vi "SensorTester.vi"() -> ()   [LabVIEW 2019]
uses:
  <vilib>/myRIO/Instrument Drivers/Onboard IO/AI/typedefs/AI Reference.ctl
  <vilib>/myRIO/Common/Instrument Driver Framework/Utilities/typedefs/myRIO Generic Hardware Reference.ctl
  <vilib>/myRIO/Common/Instrument Driver Framework/Utilities/typedefs/Hardware Version Enum.ctl
  <vilib>/myRIO/Common/Instrument Driver Framework/Utilities/typedefs/myRIO v1.0 Reference.ctl
  <vilib>/myRIO/Common/Instrument Driver Framework/Utilities/typedefs/Generic FPGA Reference.ctl
  <vilib>/myRIO/Common/Instrument Driver Framework/myRIO v1.0/AI/typedefs/AI Channels List.ctl
  <vilib>/myRIO/Common/Instrument Driver Framework/myRIO v1.0/AI/typedefs/AI Channels Enum.ctl
  <vilib>/myRIO/Common/Instrument Driver Framework/Utilities/typedefs/Analog Scaling Constants List.ctl
  <vilib>/myRIO/Common/Instrument Driver Framework/Utilities/typedefs/Analog Scaling Constants.ctl
  <vilib>/userDefined/High Color/nirio_resource_hc.ctl
  <vilib>/myRIO/Instrument Drivers/Onboard IO/PWM/typedefs/PWM Reference.ctl
  <vilib>/myRIO/Common/Instrument Driver Framework/myRIO v1.0/PWM/typedefs/PWM Channels Enum.ctl
  <vilib>/myRIO/Instrument Drivers/Onboard IO/PWM/typedefs/PWM Configuration.ctl
  <vilib>/myRIO/Common/Instrument Driver Framework/Utilities/vis/Is FPGA Ref Available.vi
  <vilib>/myRIO/Common/Instrument Driver Framework/myRIO v1.0/AI/vis/myRIO v1.1 Open AI.vi
  <vilib>/myRIO/Instrument Drivers/Onboard IO/AI/vis/Read.vi
  <vilib>/myRIO/Common/Instrument Driver Framework/myRIO v1.0/PWM/vis/myRIO v1.1 Open PWM.vi
  <vilib>/myRIO/Instrument Drivers/Onboard IO/PWM/vis/Set Duty Cycle and Frequency.vi
  <vilib>/myRIO/Common/Instrument Driver Framework/Utilities/vis/Validate Channels.vi
  <vilib>/myRIO/Common/Instrument Driver Framework/myRIO v1.0/AI/vis/myRIO v1.0 Reserve AI.vi
  <vilib>/myRIO/Common/Instrument Driver Framework/myRIO v1.0/PWM/vis/myRIO v1.0 Reserve PWM.vi
  <vilib>/myRIO/Common/Instrument Driver Framework/myRIO v1.0/UART/vis/myRIO v1.0 Close UART.vi
  <vilib>/myRIO/Common/Instrument Driver Framework/myRIO v1.0/AI/vis/myRIO v1.0 Build MUX Configuration AI.vi
  <vilib>/myRIO/Common/Instrument Driver Framework/myRIO v1.0/Resource Manager/vis/myRIO v1.0 Reserve Channel List.vi
  <vilib>/myRIO/Common/Instrument Driver Framework/myRIO v1.0/PWM/vis/myRIO v1.0 Build MUX Configuration PWM.vi
  <vilib>/myRIO/Common/Instrument Driver Framework/myRIO v1.0/Resource Manager/vis/myRIO v1.0 Reserve Channel.vi
  <vilib>/myRIO/Common/Instrument Driver Framework/myRIO v1.0/Resource Manager/vis/myRIO v1.0 Unreserve Channel.vi
  <vilib>/myRIO/Common/Instrument Driver Framework/myRIO v1.0/Resource Manager/vis/myRIO v1.0 Create Configuration List.vi
  <vilib>/myRIO/Common/Instrument Driver Framework/myRIO v1.0/Resource Manager/vis/myRIO v1.0 Build Mutex Name.vi
  <vilib>/Utility/VariantDataType/GetNumericInfo.vi
  <vilib>/Utility/error.llb/Error Cluster From Error Code.vi
  <vilib>/myRIO/Common/Instrument Driver Framework/myRIO v1.0/myRIO v1.1 Open.vi
  <vilib>/myRIO/Common/Instrument Driver Framework/myRIO v1.0/AI/vis/myRIO v1.0 Get Scaling Constants AI.vi
  <vilib>/myRIO/Common/Instrument Driver Framework/Utilities/vis/IO Manager.vi
  <vilib>/myRIO/Common/Instrument Driver Framework/Utilities/vis/Configuration Manager.vi
  <vilib>/myRIO/Common/Instrument Driver Framework/myRIO v1.0/myRIO v1.0 Close.vi
  <vilib>/myRIO/Common/Instrument Driver Framework/myRIO v1.0/AI/vis/myRIO v1.0 Read AI.vi
  <vilib>/imath/engines/lvmath2/RunTimeEngine/Managers/WorkSpace/UID Generator.vi
  <vilib>/imath/engines/lvmath2/RunTimeEngine/RunTimeType/NIMS_RunTimeType_From StrictType (excl LVString).vi
  <instcachedir>/0/NIMS_RunTimeType_From StrictType (excl LVString)_D8AFBA86A94845AAA577C895450664BD.lvgen/NIMS_RunTimeType_From StrictType (excl LVString)_D8AFBA86A94845AAA577C895450664BD_000.vi
  <vilib>/imath/engines/lvmath2/RunTimeEngine/LocalVariableDefStatement/MC_LocalVariableDefStatement_Display.vi
  <vilib>/imath/engines/lvmath2/RunTimeEngine/Managers/SymbolTable/Clear UID.vi
  <vilib>/imath/engines/lvmath2/RunTimeEngine/NodeEndStatement/NIMS_NodeEndStatement_Output.vi
  <instcachedir>/0/NIMS_NodeEndStatement_Output_53EC0D466D134D7ABD903AC30B43404B.lvgen/NIMS_NodeEndStatement_Output_53EC0D466D134D7ABD903AC30B43404B_001.vi
  <vilib>/imath/engines/lvmath2/RunTimeEngine/ErrorHandling/NIMS_Finalize Error.vi
  <vilib>/addons/control/pid/pid.llb/PID (DBL).vi
  <vilib>/myRIO/Common/Instrument Driver Framework/myRIO v1.0/Resource Manager/vis/myRIO v1.0 Configure IO.vi
  <vilib>/myRIO/Common/Instrument Driver Framework/myRIO v1.0/PWM/vis/myRIO v1.0 Write PWM.vi
  <vilib>/myRIO/Common/Instrument Driver Framework/Utilities/vis/FPGA Ref Manager.vi
  <vilib>/myRIO/Common/Instrument Driver Framework/myRIO v1.0/myRIO v1.0 Reset FPGA.vi
  <vilib>/myRIO/Common/Instrument Driver Framework/myRIO v1.0/IRQ/vis/myRIO v1.0 IRQ Info FGV.vi
  <vilib>/myRIO/Common/Instrument Driver Framework/myRIO v1.0/IRQ/vis/myRIO v1.0 Timer IRQ Info FGV.vi
  <vilib>/myRIO/Common/Instrument Driver Framework/myRIO v1.0/IRQ/vis/myRIO v1.0 ISR Agent.vi
  <vilib>/myRIO/Instrument Drivers/Utilities/vis/Reset Index.vi
  <vilib>/myRIO/Common/Instrument Driver Framework/myRIO v1.0/Resource Manager/vis/myRIO v1.0 Block Write Resource Manager.vi
  <vilib>/myRIO/Express VI/Onboard IO/AI/AI Express VI.xnode
  <vilib>/myRIO/Instrument Drivers/Onboard IO/AI/vis/myRIO AI Open.xnode
  <vilib>/myRIO/Express VI/Onboard IO/PWM/PWM Express VI.xnode
  <vilib>/myRIO/Instrument Drivers/Onboard IO/PWM/vis/myRIO PWM Open.xnode
  <vilib>/myRIO/Instrument Drivers/Onboard IO/PWM/PWM.lvlib
  <vilib>/myRIO/Instrument Drivers/Onboard IO/AI/AI.lvlib
  <vilib>/imath/engines/lvmath2/RunTimeEngine/Managers/SymbolTable/NIMS_WorkSpace.lvlib
  <vilib>/addons/control/pid/NI_PID_pid.lvlib
  <vilib>/ptbypt/NI_PtbyPt.lvlib
  <vilib>/myRIO/Instrument Drivers/Utilities/Utilities.lvlib
panel:
  out "VA_sensor 6":dbl format="%#.3g"
  out "VA_sensor 5":dbl format="%#.3g"
  out "VA_sensor 4":dbl format="%#.3g"
  out "VA_sensor 3":dbl format="%#.3g"
  out "VA_sensor 2":dbl format="%#.3g"
  in  "stop":bool
  out "VA_sensor":dbl format="%#.3g"
  out "Pressures Receiver":cluster{dbl, dbl}(knob)={0.0, 8.870406975580165} scale=0.0..120.0
  in  "Setpoint Preceiver":dbl(slide) scale=0.0..100.0
  out "V_Rsensor":dbl format="%#.3g"
  in  "PID Motor":T1={"proportional gain (Kc)"=0.01, "integral time (Ti, min)"=0.005, "derivative time (Td, min)"=0.0} {"derivative time (Td, min)" format="%.3f"; "integral time (Ti, min)" format="%.3f"; "proportional gain (Kc)" format="%.3f"}
  out "Duty cycle Motor":dbl(knob) scale=0.0..1.0
  out "Pressures Actuator":dynamicdata(graph)
  in  "milliseconds to wait":u32=100
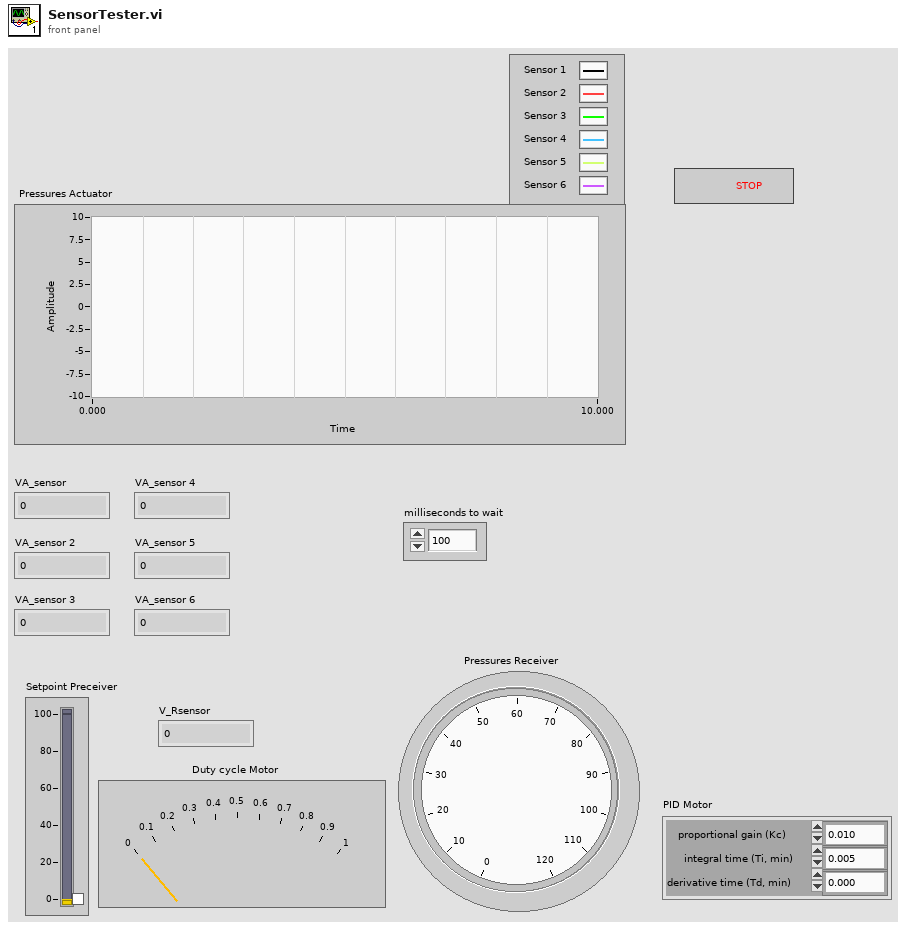
[diagram p1: front panel]
types:
  T1 = cluster{"proportional gain (Kc)":dbl, "integral time (Ti, min)":dbl, "derivative time (Td, min)":dbl}
  T2 = typedef "AI.lvlib/AI Reference.ctl" = cluster{"myRIO Reference":T3, "AI Channels List":T7, "AI Scaling Constants List":T9}
  T3 = typedef "myRIO Generic Hardware Reference.ctl" = cluster{"myRIO Model":T4, "myRIO Hardware Reference":T5}
  T4 = typedef "Hardware Version Enum.ctl" = enum16{"Unknown", "myRIO-1900", "myRIO-1950", "roboRIO", "NI ELVIS RIO CM", "ELVIS III"}
  T5 = typedef "myRIO v1.0 Reference.ctl" = cluster{"Generic FPGA Reference":T6, "Allow multiple opens":bool}
  T6 = typedef "Generic FPGA Reference.ctl" = refnum<k20>
  T7 = typedef "AI Channels List.ctl" = T8[]
  T8 = typedef "AI Channels Enum.ctl" = enum16{"Not Connected", "AudioIn/Left", "AudioIn/Right", "C/AI0", "C/AI1", "A/AI0", "A/AI1", "A/AI2", "A/AI3", "A/AI4", "A/AI5", "A/AI6", "A/AI7", "B/AI0", "B/AI1", "B/AI2", "B/AI3", "B/AI4", "B/AI5", "B/AI6", "B/AI7", "AI/AI0", "AI/AI1", "AI/AI2", "AI/AI3", "A/AI0 (DIFF)", "A/AI1 (DIFF)", "A/AI2 (DIFF)", "A/AI3 (DIFF)", "B/AI0 (DIFF)", "B/AI1 (DIFF)", "B/AI2 (DIFF)", "B/AI3 (DIFF)"}
  T9 = typedef "Analog Scaling Constants List.ctl" = T10[]
  T10 = typedef "Analog Scaling Constants.ctl" = cluster{"LSB Weight (Volts)":dbl, "Offset (Volts)":dbl, "Signed?":bool}
  T11 = typedef "nirio_resource_hc.ctl" = tag
  T12 = typedef "PWM.lvlib/PWM Reference.ctl" = cluster{"myRIO Reference":T3, "PWM Channels Enum":T13, "PWM Configuration":T14}
  T13 = typedef "PWM Channels Enum.ctl" = enum16{"Not Connected", "C/PWM0", "C/PWM1", "A/PWM0", "A/PWM1", "A/PWM2", "A/PWM3", "A/PWM4", "A/PWM5", "A/PWM6", "A/PWM7", "A/PWM8", "A/PWM9", "A/PWM10", "A/PWM11", "A/PWM12", "A/PWM13", "A/PWM14", "A/PWM15", "A/PWM16", "A/PWM17", "A/PWM18", "A/PWM19", "B/PWM0", "B/PWM1", "B/PWM2", "B/PWM3", "B/PWM4", "B/PWM5", "B/PWM6", "B/PWM7", "B/PWM8", "B/PWM9", "B/PWM10", "B/PWM11", "B/PWM12", "B/PWM13", "B/PWM14", "B/PWM15", "B/PWM16", "B/PWM17", "B/PWM18", "B/PWM19", "PWM/PWM0", "PWM/PWM1", "PWM/PWM2", "PWM/PWM3", "PWM/PWM4", "PWM/PWM5", "PWM/PWM6", "PWM/PWM7", "PWM/PWM8", "PWM/PWM9"}
  T14 = typedef "PWM.lvlib/PWM Configuration.ctl" = cluster{"Frequency":dbl, "Duty Cycle":dbl}
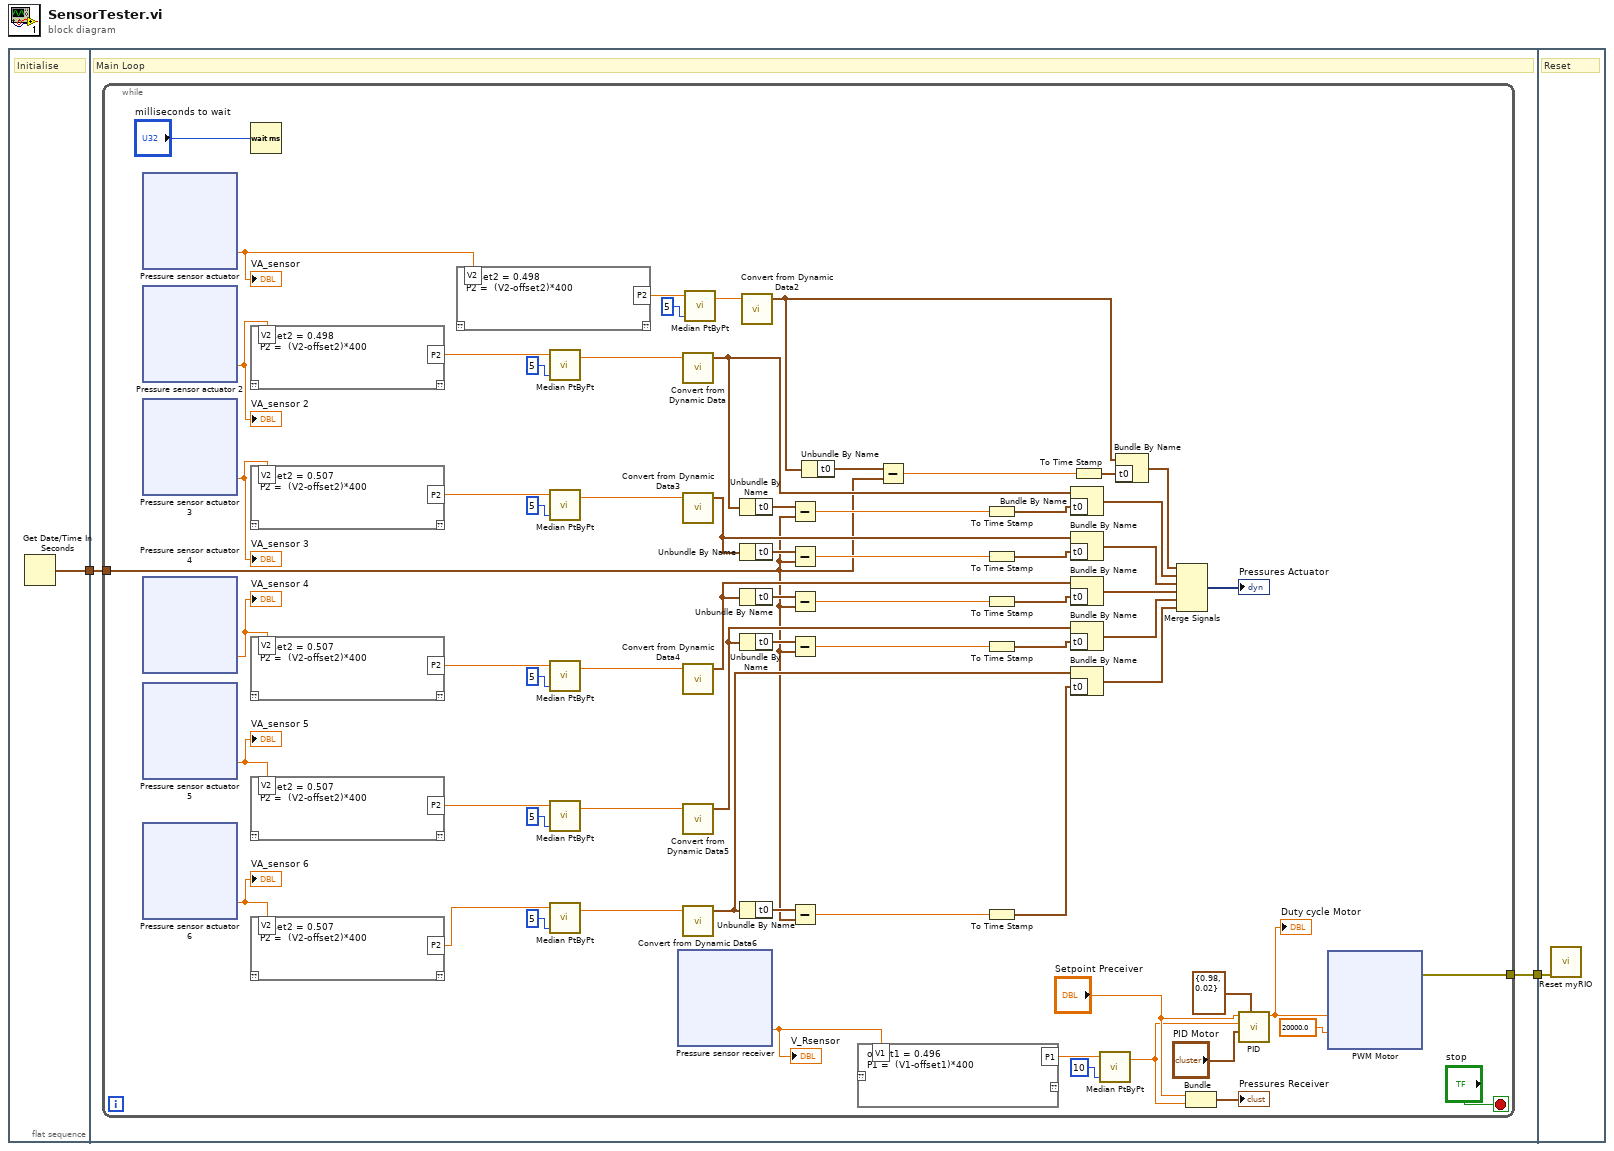
[diagram p0: block diagram]
diagram:
  n1 = flat-sequence {
    tunnel: [w3] -> w2
    tunnel: [w5] -> w1
    tunnel: w2 -> [w4]
    tunnel: w1 -> [w726]
    frame #0 {
      # "Initialise"
      n2 = Get Date/Time In Seconds() -> (seconds since 1Jan1904=w3:timestamp)
    }
    frame #1 {
      # "Main Loop"
      n3 = while {
        tunnel: [w64] -> w5
        tunnel: w4 -> [w33]
        stop <- "stop" stop-if-true
        n4 = xnode "Pressure sensor actuator"() -> ("B/AI1 (Pin 5)"=w11:dbl)  [unwired: 1 in, 1 out]
        "VA_sensor" <- w11
        n5 = xnode "Pressure sensor actuator 2"() -> ("B/AI2 (Pin 7)"=w10:dbl)  [unwired: 1 in, 1 out]
        "VA_sensor 2" <- w10
        n6 = xnode "Pressure sensor actuator 3"() -> ("B/AI3 (Pin 9)"=w9:dbl)  [unwired: 1 in, 1 out]
        "VA_sensor 3" <- w9
        n7 = xnode "Pressure sensor actuator 4"() -> ("A/AI0 (Pin 3)"=w28:dbl)  [unwired: 1 in, 1 out]
        "VA_sensor 4" <- w28
        n8 = xnode "Pressure sensor actuator 5"() -> ("A/AI1 (Pin 5)"=w8:dbl)  [unwired: 1 in, 1 out]
        "VA_sensor 5" <- w8
        n9 = xnode "Pressure sensor actuator 6"() -> ("A/AI2 (Pin 7)"=w7:dbl)  [unwired: 1 in, 1 out]
        "VA_sensor 6" <- w7
        n10 = Wait (ms)(milliseconds to wait="milliseconds to wait") -> ()  [unwired: 1 out]
        n11 = mathscript code="offset2 = 0.498\nP2 =  (V2-offset2)*400"("V2"=w10) -> ("P2"=w32:dbl)  [unwired: 1 in, 1 out]
        n12 = mathscript code="offset2 = 0.507\nP2 =  (V2-offset2)*400"("V2"=w9) -> ("P2"=w30:dbl)  [unwired: 1 in, 1 out]
        n13 = mathscript code="offset2 = 0.507\nP2 =  (V2-offset2)*400"("V2"=w28) -> ("P2"=w27:dbl)  [unwired: 1 in, 1 out]
        n14 = mathscript code="offset2 = 0.507\nP2 =  (V2-offset2)*400"("V2"=w8) -> ("P2"=w25:dbl)  [unwired: 1 in, 1 out]
        n15 = mathscript code="offset2 = 0.507\nP2 =  (V2-offset2)*400"("V2"=w7) -> ("P2"=w23:dbl)  [unwired: 1 in, 1 out]
        n16 = mathscript code="offset2 = 0.498\nP2 =  (V2-offset2)*400"("V2"=w11) -> ("P2"=w74:dbl)  [unwired: 1 in, 1 out]
        n17 = call <vilib>:"Median PtByPt.vi"("sample length"=5, "x"=w32) -> ("median"=w16:dbl)  [unwired: 2 in, 1 out]
        n18 = call <vilib>:"Median PtByPt.vi"("sample length"=5, "x"=w30) -> ("median"=w15:dbl)  [unwired: 2 in, 1 out]
        n19 = call <vilib>:"Median PtByPt.vi"("sample length"=5, "x"=w27) -> ("median"=w14:dbl)  [unwired: 2 in, 1 out]
        n20 = call <vilib>:"Median PtByPt.vi"("sample length"=5, "x"=w25) -> ("median"=w13:dbl)  [unwired: 2 in, 1 out]
        n21 = call <vilib>:"Median PtByPt.vi"("sample length"=5, "x"=w23) -> ("median"=w12:dbl)  [unwired: 2 in, 1 out]
        n22 = xnode "Pressure sensor receiver"() -> ("B/AI0 (Pin 3)"=w6:dbl)  [unwired: 1 in, 1 out]
        "V_Rsensor" <- w6
        n23 = call "Convert from Dynamic Data"("Dynamic Data Type"=w16) -> ("Waveform"=w62:waveform(dbl))  [unwired: 3 in]
        n24 = call "Convert from Dynamic Data3"("Dynamic Data Type"=w15) -> ("Waveform"=w49:waveform(dbl))  [unwired: 3 in]
        n25 = call "Convert from Dynamic Data4"("Dynamic Data Type"=w14) -> ("Waveform"=w45:waveform(dbl))  [unwired: 3 in]
        n26 = call "Convert from Dynamic Data5"("Dynamic Data Type"=w13) -> ("Waveform"=w41:waveform(dbl))  [unwired: 3 in]
        n27 = call "Convert from Dynamic Data6"("Dynamic Data Type"=w12) -> ("Waveform"=w37:waveform(dbl))  [unwired: 3 in]
        n28 = call <vilib>:"Median PtByPt.vi"("sample length"=5, "x"=w74) -> ("median"=w17:dbl)  [unwired: 2 in, 1 out]
        n29 = Unbundle By Name(w62) -> ("t0"=w57:timestamp)
        n30 = Unbundle By Name(w49) -> ("t0"=w46:timestamp)
        n31 = Unbundle By Name(w45) -> ("t0"=w42:timestamp)
        n32 = Unbundle By Name(w41) -> ("t0"=w38:timestamp)
        n33 = Unbundle By Name(w37) -> ("t0"=w34:timestamp)
        n34 = call "Convert from Dynamic Data2"("Dynamic Data Type"=w17) -> ("Waveform"=w56:waveform(dbl))  [unwired: 3 in]
        n35 = Subtract(x=w57, y=w33) -> (x-y=w61:dbl)
        n36 = Subtract(x=w46, y=w33) -> (x-y=w48:dbl)
        n37 = Subtract(x=w42, y=w33) -> (x-y=w44:dbl)
        n38 = Subtract(x=w38, y=w33) -> (x-y=w40:dbl)
        n39 = Subtract(x=w34, y=w33) -> (x-y=w36:dbl)
        n40 = Unbundle By Name(w56) -> ("t0"=w53:timestamp)
        n41 = mathscript code="offset1 = 0.496\nP1 =  (V1-offset1)*400"("V1"=w6) -> ("P1"=w66:dbl)  [unwired: 1 in, 1 out]
        n42 = Subtract(x=w53, y=w33) -> (x-y=w55:dbl)
        n43 = To Time Stamp(1:w61) -> (0:w60:timestamp)
        n44 = To Time Stamp(1:w48) -> (0:w47:timestamp)
        n45 = To Time Stamp(1:w44) -> (0:w43:timestamp)
        n46 = To Time Stamp(1:w40) -> (0:w39:timestamp)
        n47 = To Time Stamp(1:w36) -> (0:w35:timestamp)
        n48 = Bundle By Name(cluster=w62, "t0"=w60) -> (w58:waveform(dbl))
        n49 = Bundle By Name(cluster=w49, "t0"=w47) -> (w21:waveform(dbl))
        n50 = Bundle By Name(cluster=w45, "t0"=w43) -> (w20:waveform(dbl))
        n51 = Bundle By Name(cluster=w41, "t0"=w39) -> (w19:waveform(dbl))
        n52 = Bundle By Name(cluster=w37, "t0"=w35) -> (w18:waveform(dbl))
        n53 = To Time Stamp(1:w55) -> (0:w54:timestamp)
        n54 = call <vilib>:"Median PtByPt.vi"("sample length"=10, "x"=w66) -> ("median"=w68:dbl)  [unwired: 2 in, 1 out]
        n55 = Bundle By Name(cluster=w56, "t0"=w54) -> (w52:waveform(dbl))
        n56 = Merge Signals(w52, w58, w21, w20, w19, w18) -> (→"Pressures Actuator":dynamicdata)
        n57 = Bundle("Setpoint Preceiver"="Setpoint Preceiver", "median"=w68) -> (→"Pressures Receiver":cluster{"Setpoint Preceiver":dbl, "median":dbl})  [unwired: 1 in]
        n58 = call-poly <vilib>:"PID.vi"("output range"=cluster{"output high":dbl, "output low":dbl} {"output high"=0.98, "output low"=0.02} ("output range motor"), "PID gains"="PID Motor", "process variable"=w68, "setpoint"="Setpoint Preceiver") -> ("output"=w63:dbl)  [unwired: 6 in, 1 out]
        "Duty cycle Motor" <- w63
        n59 = xnode "PWM Motor"("Duty Cycle"=w63, "Frequency [Hz]"=20000.0) -> ("error out"=w64:errorcluster)  [unwired: 1 in]
      }
    }
    frame #2 {
      # "Reset"
      n60 = call <vilib>:"Reset myRIO.vi"("error in (no error)"=w726) -> ()  [unwired: 10 in, 1 out]
    }
  }
